vi "Init Actor Default.vi"() -> (2 "Actor":refnum<class "Actor.lvclass">)   [LabVIEW 2025, in "_Template.lvlib" / "Templates.lvlib" / "TEMPLATE jettl Actor.lvlib" / "TEMPLATE.lvlib"]
uses:
  TEMPLATE.lvlib
  jettl/jettl/Actor/Actor.lvclass
  TEMPLATE Actor/TEMPLATE Actor.lvlib
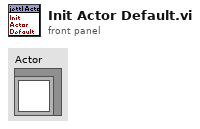
[diagram p1: front panel]
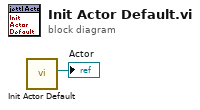
[diagram p0: block diagram]
diagram:
  n1 = call "Init Actor Default.vi"() -> ("Actor"=→"Actor":refnum<class "Actor.lvclass">)  [unwired: 11 in]
